vi "SetTriggerInputLine.vi"(8 "Error In":errorcluster, 10 "Line (1-6)":u8=1 min=1 step=1, 11 "Keithley 6482 In":refnum<visa-resource-name>) -> (0 "Error Out":errorcluster, 3 "Keithley 6482 Out":refnum<visa-resource-name>)   [LabVIEW 2014, in "Keithley-6482-Visa.lvlib"]
uses:
  Keithley-6482-Visa.lvlib
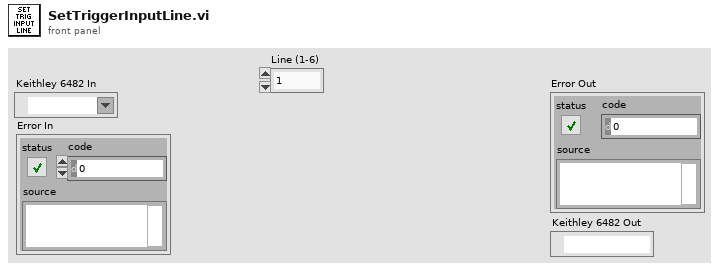
[diagram p1: front panel]
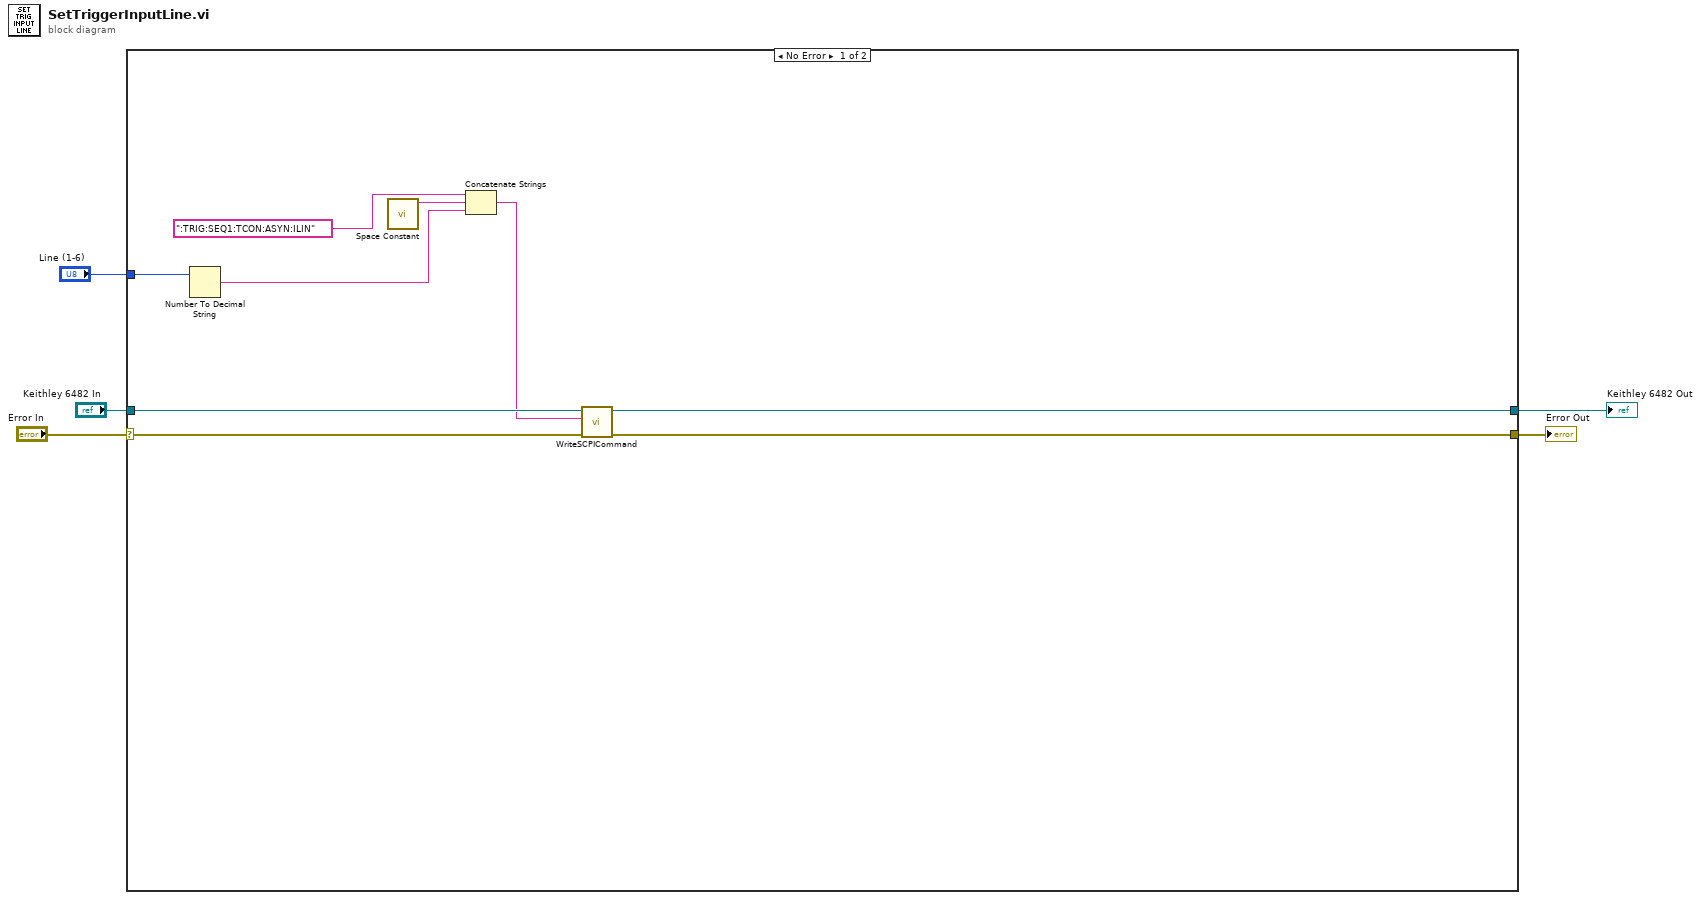
[diagram p0: block diagram]
diagram:
  n1 = case shown="No Error" "Error In" {
    selector: "Error In" -> [w14 w15]
    tunnel: "Keithley 6482 In" -> [w13 w16]
    tunnel: [w8 w15] -> w3
    tunnel: [w9 w16] -> w2
    tunnel: "Line (1-6)" -> [w7 _]
    frame No Error {
      n2 = Number To Decimal String(number=w7) -> (decimal integer string=w6:string)  [unwired: 1 in]
      n3 = call <vilib>:"Space Constant.vi"() -> ("String"=w11:string)
      n4 = Concatenate Strings(":TRIG:SEQ1:TCON:ASYN:ILIN" ("string"), w11, w6) -> (w10:string)
      n5 = call "WriteSCPICommand.vi"("Error In"=w14, "SCPI Command"=w10, "Keithley 6482 In"=w13) -> ("Error Out"=w8:errorcluster, "Keithley 6482 Out"=w9:refnum<visa-resource-name>)  [unwired: 7 in]
    }
    frame Error {
    }
  }
  "Error Out" <- w3
  "Keithley 6482 Out" <- w2
